vi "OCT Bscan Test_3.vi"() -> ()   [LabVIEW 2017]
panel:
  in  "Boolean":bool=TRUE
  out "Intensity Graph":dbl[][](graph)
  out "error out":errorcluster
  in  "Objective":u16(ring)=1 items=["5X LKM05", "10X LKM10", "20X LKM20", "10X LSM02"]
  in  "Scan Parameters":T1={"# Scan"={"#Ascan"=400, "#Bscan"=400}, "# Rpt"={"#ARpt"=1, "#BRpt"=1}, "Aline Rate"=2, "# Extra"={"# ARpt_extra"=5, "#Brtn_extra"=80}} {"Aline Rate" items=["76 KHz", "146 KHz", "76 KHz", "28 KHz", "10 KHz"]}
  in  "ROI Parameters":T2={"ROI (mm)"={"X (mm)"=1.0, "Y (mm)"=1.0}, "Shift (mm)"={"Xshift (mm)"=0.0, "Yshift (mm)"=0.0}}
  in  "error in":errorcluster
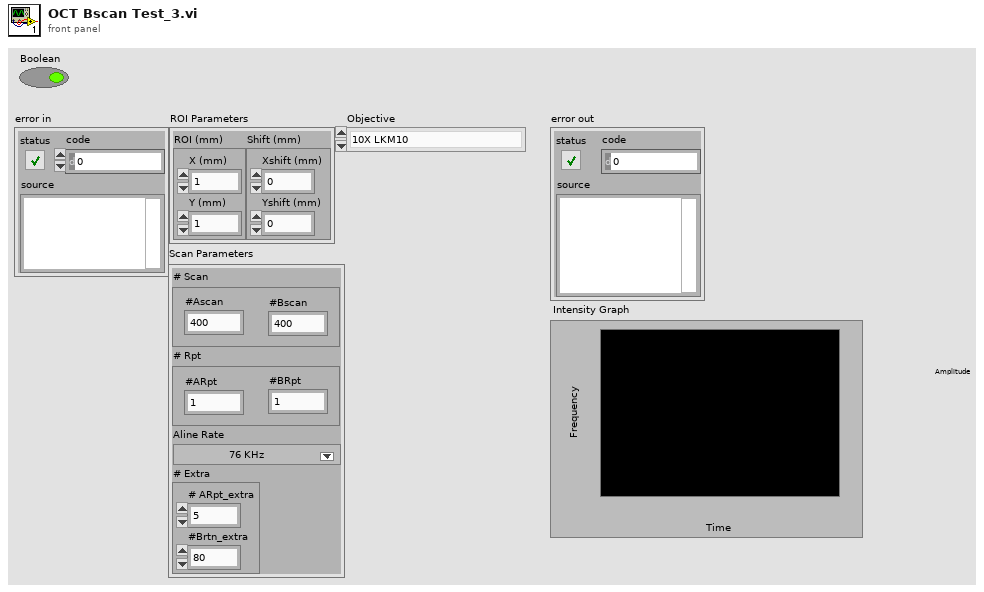
[diagram p1: front panel]
types:
  T1 = cluster{"# Scan":cluster{"#Ascan":i32, "#Bscan":i32}, "# Rpt":cluster{"#ARpt":i32, "#BRpt":i32}, "Aline Rate":u16, "# Extra":cluster{"# ARpt_extra":i32, "#Brtn_extra":i32}}
  T2 = cluster{"ROI (mm)":cluster{"X (mm)":sgl, "Y (mm)":sgl}, "Shift (mm)":cluster{"Xshift (mm)":sgl, "Yshift (mm)":sgl}}
  T3 = enum16{"Init", "Configure", "Configure Data", "Generate Scan Pattern", "Start Acquire Raw", "Start Acquire Data", "Acquire RAW", "Acquire Data", "Stop Acquire", "Uninit"}
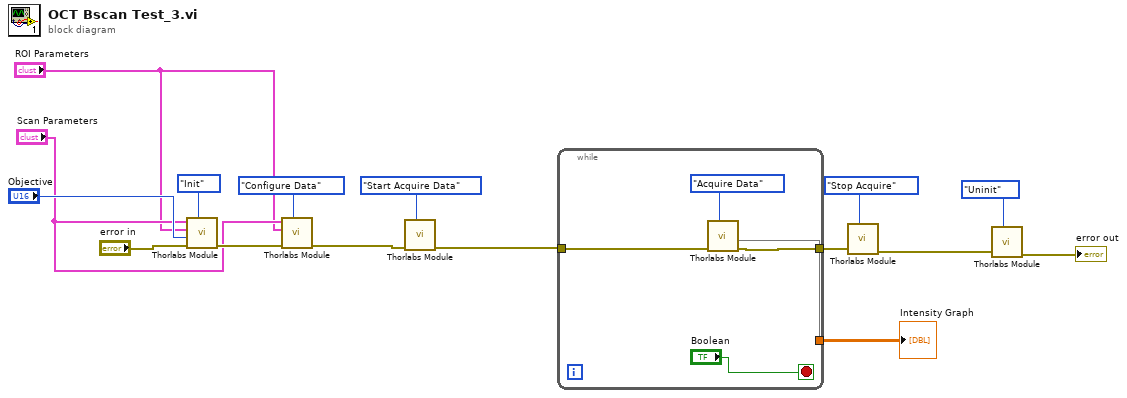
[diagram p0: block diagram]
diagram:
  n1 = call "Thorlabs Module.vi"("Actions"=T3."Init", "error in"="error in", "Objective"="Objective", "ROI Parameters"="ROI Parameters", "Scan Parameters"="Scan Parameters") -> ("error out"=w16:errorcluster)  [unwired: 4 in, 2 out]
  n2 = call "Thorlabs Module.vi"("Actions"=T3."Configure Data", "error in"=w16, "ROI Parameters"="ROI Parameters", "Scan Parameters"="Scan Parameters") -> ("error out"=w4:errorcluster)  [unwired: 5 in, 2 out]
  n3 = call "Thorlabs Module.vi"("Actions"=T3."Start Acquire Data", "error in"=w4) -> ("error out"=w3:errorcluster)  [unwired: 7 in, 2 out]
  n4 = while {
    tunnel: w3 -> [w19]
    tunnel: [w20] -> w11
    tunnel: [w17] -> w1
    stop <- "Boolean" stop-if-true
    n5 = call "Thorlabs Module.vi"("Actions"=T3."Acquire Data", "error in"=w19) -> ("error out"=w20:errorcluster, 4:w17)  [unwired: 6 in, 2 out]
  }
  "Intensity Graph" <- w1
  n6 = call "Thorlabs Module.vi"("Actions"=T3."Stop Acquire", "error in"=w11) -> ("error out"=w9:errorcluster)  [unwired: 7 in, 2 out]
  n7 = call "Thorlabs Module.vi"("Actions"=T3."Uninit", "error in"=w9) -> ("error out"=→"error out":errorcluster)  [unwired: 7 in, 2 out]
